vi "Simple Lock-in_read_test.vi"() -> ()   [LabVIEW 2020]
panel:
  in  "Tab Control":enum32{"Basic", "Advanced"}(tab)
  out "Waveform Chart":dbl[][](graph)
  in  "Number of channels #2":i32
  in  "Ranges and couplings  #2":cluster{"Range":dbl, "Coupling":i32}[](array[cluster]) {"Coupling" items=["default"=-1, "RSE"=10083, "NRSE"=10078, "Differential"=10106, "Pseudodifferential"=12529]}
  in  "AI #2 NI device":tag
  in  "AI+AO #1 NI device":tag
  in  "Ranges and couplings #1":cluster{"Range":dbl, "Coupling":i32}[](array[cluster])=[{"Range"=10.0, "Coupling"=10106}] {"Coupling" items=["default"=-1, "RSE"=10083, "NRSE"=10078, "Differential"=10106, "Pseudodifferential"=12529]}
  in  "Number of channels #1":i32=1
  in  "Sine frequency, Hz":dbl=100.0 format="%#_6p"
  in  "Sine amplitude, V":dbl=1.0 format="%0.2f"
  in  "stop":bool
  in  "dev #2 clock terminal":string="PXI_Trig0"
  in  "Samples per sine wave":i32=100
  in  "Time constant, s":dbl=1.0
  in  "Phase":dbl
  in  "Amplitude scale":enum16{"Amplitude", "RMS", "Peak-to-Peak"}(ring)
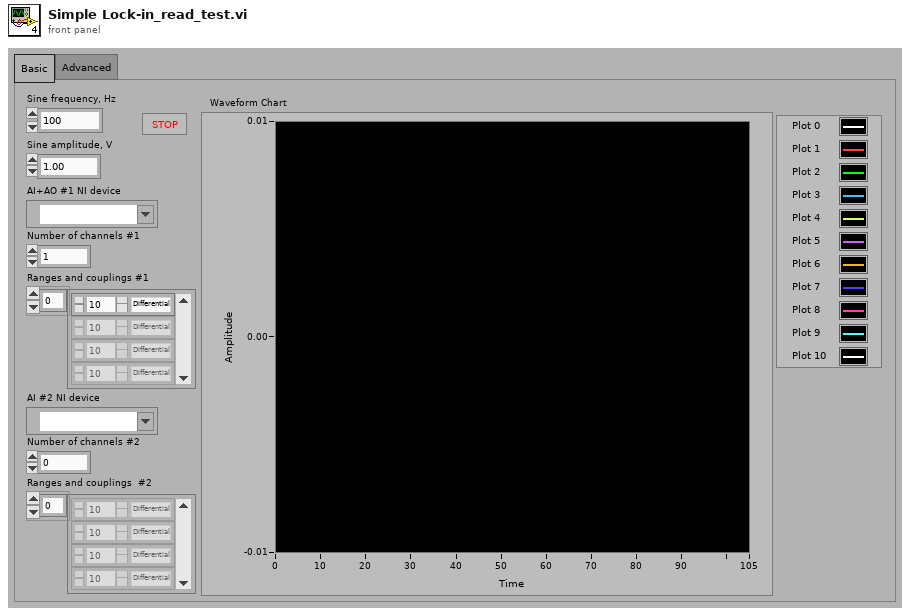
[diagram p1: front panel]
types:
  T1 = cluster{"Sine Frequency, Hz":dbl, "Post-filter\ncutoff freq, Hz":dbl, "Post-Filter type":enum16{"Butterworth", "No filtering"}, "Output Representation":enum16{"Real/Imaginary", "Polar"}, "Phase":dbl, "Post-filter Order":i32, "decimating factor":i32, "Samples to Read":i32, "Post-filter decimation":i32, "Blocks to average":i32, "Trig delay, points":i32}
  T2 = cluster{"Sample clock source":string, "Sample mode":i32, "Sample clock rate":dbl, "Samples per channel":i32, "Trigger type":enum16{"Reference", "Immediate", "Start"}, "Trigger source":string, "Pretrigger samples":u32}
  T3 = typedef "Lockin Settings.ctl" = cluster{"Sine Frequency, Hz":dbl, "Time constant, s":dbl, "Low-pass filter":enum16{"No filtering", "Butterworth", "Bessel"}, "Output representation":enum16{"Real/Imaginary", "Polar"}, "Phases, deg":dbl[], "Low-pass filter Order":i32, "Decimating factor":i32, "Samples to Read":i32, "Post-filter decimation":i32, "Blocks to average":i32, "Trig delay, points":i32, "Harmonics per channel":T4, "Amplitude scale":enum16{"Amplitude", "RMS", "Peak-to-Peak"}}
  T4 = typedef "Harmonics per channel.ctl" = cluster{"Harmonics":i32[]}[]
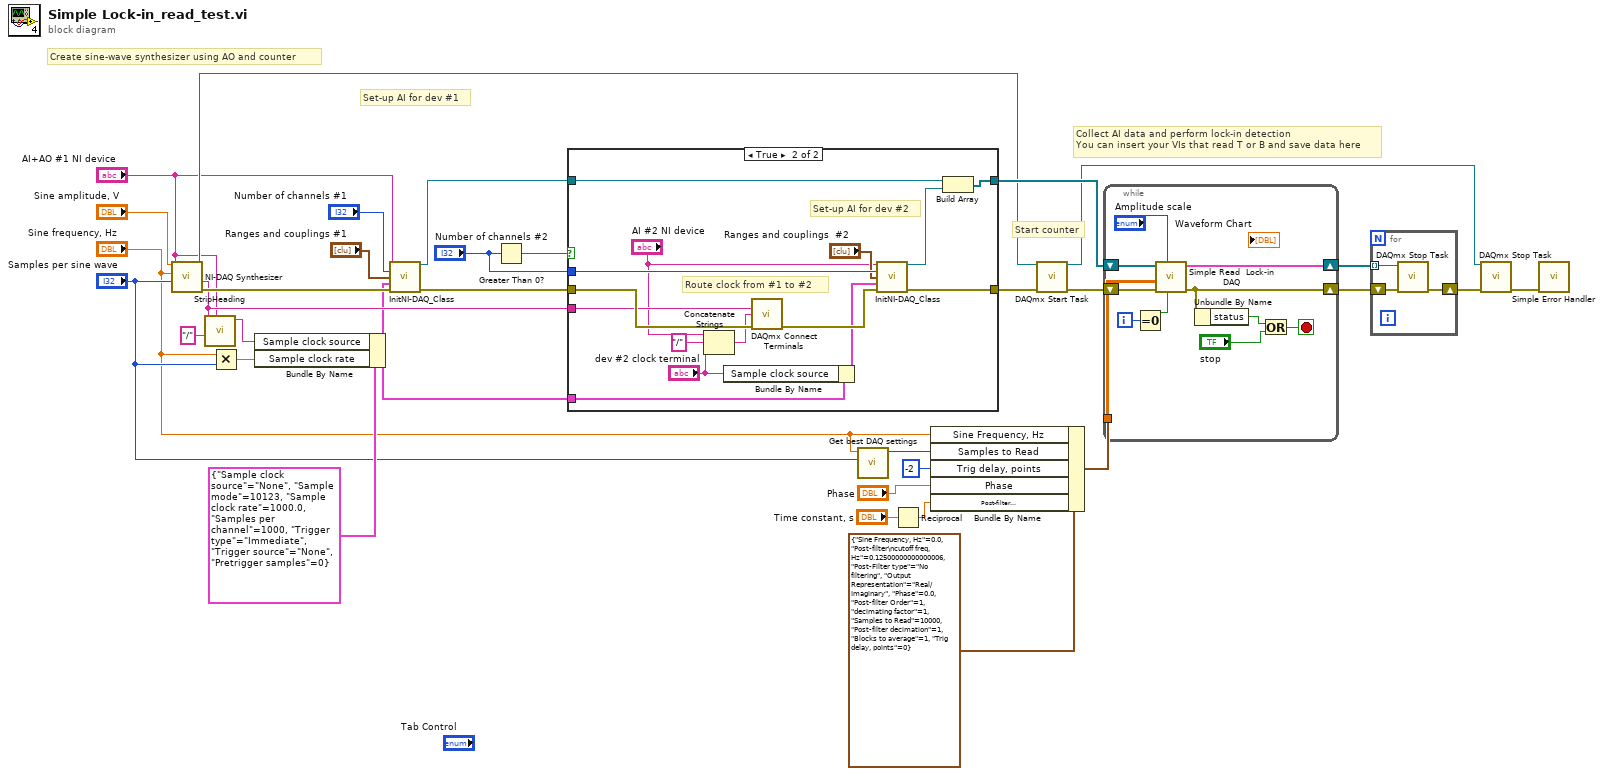
[diagram p0: block diagram]
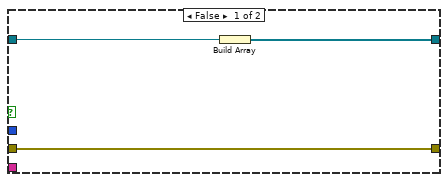
[diagram p2: hidden frame]
diagram:
  # "Collect AI data and perform lock-in detection\nYou can insert your VIs that read T or B and save data here"
  # "Start counter"
  # "Set-up AI for dev #1"
  # "Create sine-wave synthesizer using AO and counter"
  n1 = call "NI-DAQ Synthesizer.vi"("Amplitude, V"="Sine amplitude, V", "Samples per sine wave"="Samples per sine wave", "Sine frequency, Hz"="Sine frequency, Hz", "DAQmx Device Name"="AI+AO #1 NI device") -> ("error out"=w29:errorcluster, "DAQ Clock channel name"=w8:string, "Counter task out"=w13:refnum<k21>)  [unwired: 4 in, 1 out]
  n2 = call "StripHeading.vi"("Header"="AI+AO #1 NI device", "Padding"="/", "Resource in"=w8) -> ("Resource out"=w9:string)  [unwired: 8 in]
  n3 = Multiply(x="Sine frequency, Hz", y="Samples per sine wave") -> (x*y=w23:dbl)
  n4 = Bundle By Name(cluster=T2 {"Sample clock source"="None", "Sample mode"=10123, "Sample clock rate"=1000.0, "Samples per channel"=1000, "Trigger type"=enum."Immediate", "Trigger source"="None", "Pretrigger samples"=0} ("Clock and trigger"), "Sample clock source"=w9, "Sample clock rate"=w23) -> (w4:T2)
  n5 = call "InitNI-DAQ_Class.vi"("DAQmx Device Name"="AI+AO #1 NI device", "Number of channels"="Number of channels #1", "Ranges and couplings"="Ranges and couplings #1", "Clock and trigger"=w4, "error in (no error)"=w29) -> ("task out"=w25:refnum<k21>, "error out"=w30:errorcluster)  [unwired: 9 in]
  n6 = Greater Than 0?(x="Number of channels #2") -> (x > 0?=w27:bool)
  n7 = case shown="True" w27 {
    tunnel: w30 -> [w36 w46]
    tunnel: "Number of channels #2" -> [_ w51]
    tunnel: [w36 w50] -> w22
    tunnel: w25 -> [w34 w49]
    tunnel: [w35 w47] -> w17
    tunnel: w8 -> [_ w44]
    tunnel: w4 -> [_ w40]
    frame False {
      n8 = Build Array(w34) -> (w35:refnum<k21>[])
    }
    frame True {
      # "Route clock from #1 to #2"
      # "Set-up AI for dev #2"
      n9 = Concatenate Strings("AI #2 NI device", "/" ("string"), "dev #2 clock terminal") -> (w42:string)
      n10 = Bundle By Name(cluster=w40, "Sample clock source"="dev #2 clock terminal") -> (w41:T2)
      n11 = call <vilib>:"DAQmx Connect Terminals.vi"("source terminal"=w44, "destination terminal"=w42, "error in"=w46) -> ("error out"=w45:errorcluster)  [unwired: 12 in]
      n12 = call "InitNI-DAQ_Class.vi"("DAQmx Device Name"="AI #2 NI device", "Number of channels"=w51, "Ranges and couplings"="Ranges and couplings  #2", "Clock and trigger"=w41, "error in (no error)"=w45) -> ("task out"=w48:refnum<k21>, "error out"=w50:errorcluster)  [unwired: 9 in]
      n13 = Build Array(w49, w48) -> (w47:refnum<k21>[])
    }
  }
  n14 = call "Get best DAQ settings.vi"("Samples per sine wave"="Samples per sine wave", "Sine frequency, Hz"="Sine frequency, Hz") -> ("Samples per read"=w18:i32)  [unwired: 9 in]
  n15 = Reciprocal(x="Time constant, s") -> (1/x=w1:dbl)
  n16 = Bundle By Name(cluster=T1 {"Sine Frequency, Hz"=0.0, "Post-filter\ncutoff freq, Hz"=0.12500000000000006, "Post-Filter type"=enum."No filtering", "Output Representation"=enum."Real/Imaginary", "Phase"=0.0, "Post-filter Order"=1, "decimating factor"=1, "Samples to Read"=10000, "Post-filter decimation"=1, "Blocks to average"=1, "Trig delay, points"=0} ("Lock-in settings"), "Sine Frequency, Hz"="Sine frequency, Hz", "Samples to Read"=w18, "Trig delay, points"=-2, "Phase"="Phase", "Post-filter\ncutoff freq, Hz"=w1) -> (w20:T1)
  n17 = call <vilib>:"DAQmx Start Task.vi"("task/channels in"=w13, "error in"=w22) -> ("task out"=w11:refnum<k21>, "error out"=w14:errorcluster)  [unwired: 12 in]
  n18 = while {
    tunnel: w20 -> [w61]
    shift-right: [w56] -> w16
    shift-left: w14 -> [w62]
    shift-right: [w57] -> w15
    shift-left: w17 -> [w60]
    i -> [w59]
    stop <- w53 stop-if-true
    n19 = Equal To 0?(x=w59) -> (x = 0?=w58:bool)
    n20 = call "Simple Read  Lock-in DAQ.vi"("Raw data"=w58, "Initialize?"="Amplitude scale", "error in (no error)"=w62, "Lock-in settings"=w60) -> ("error out"=w56:errorcluster, "Lock-in settings out"=w57:T3, "signal(s) out"=w61:dbl[][])  [unwired: 2 in, 3 out]
    n21 = Unbundle By Name(w56) -> ("status"=w55:bool)
    n22 = Or(x=w55, y="stop") -> (x .or. y?=w53:bool)
  }
  n23 = for {
    tunnel: w15 -> [w64] mode=indexing
    shift-right: [w63] -> w12
    shift-left: w16 -> [w65]
    n24 = call <vilib>:"DAQmx Stop Task.vi"("task/channels in"=w64, "error in"=w65) -> ("error out"=w63:errorcluster)  [unwired: 12 in, 1 out]
  }
  n25 = call <vilib>:"DAQmx Stop Task.vi"("task/channels in"=w11, "error in"=w12) -> ("error out"=w10:errorcluster)  [unwired: 12 in, 1 out]
  n26 = call <vilib>:"Simple Error Handler.vi"("error in (no error)"=w10) -> ()  [unwired: 4 in, 5 out]
